vi "Trigger Ref DB (eFGV).vi"(7 "Action":T1, 8 "error in":errorcluster, 11 "Data In":bool) -> (0 "error out":errorcluster, 2 "ref":refnum<user-event>, 3 "Data out":bool)   [LabVIEW 2019]
uses:
  Controls/eFGV States.ctl
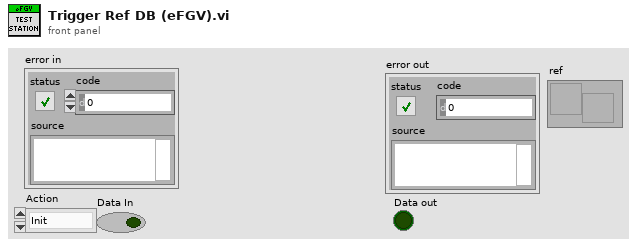
[diagram p1: front panel]
types:
  T1 = typedef "eFGV States.ctl" = enum16{"Init", "Read", "Write", "Exit"}
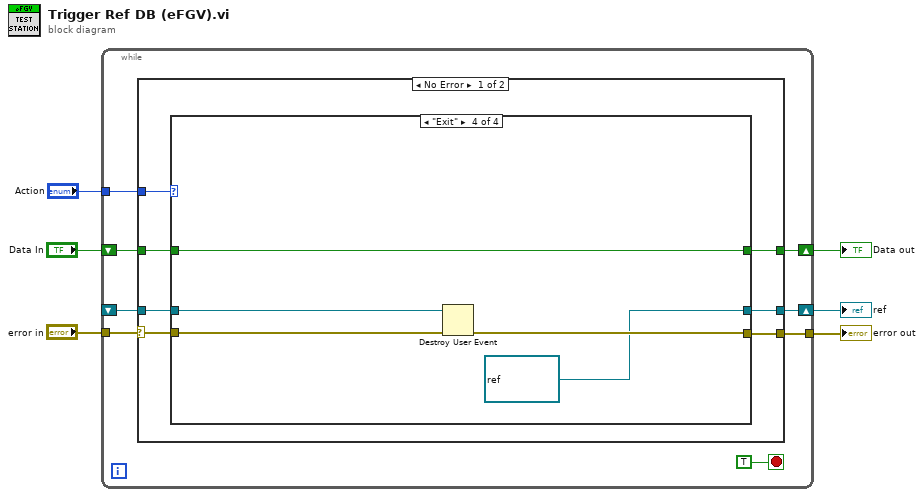
[diagram p0: block diagram]
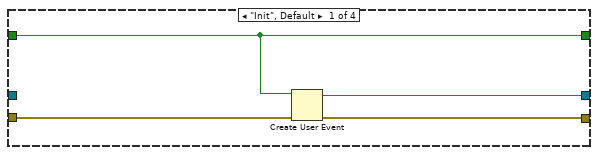
[diagram p2: hidden frame]
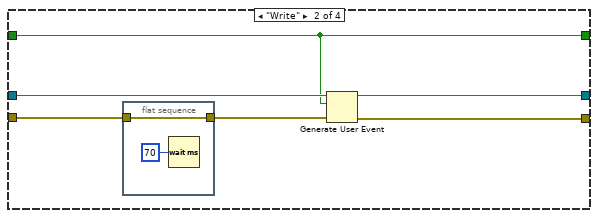
[diagram p3: hidden frame]
diagram:
  n1 = while {
    tunnel: "Action" -> [w11]
    tunnel: "error in" -> [w13]
    tunnel: [w12] -> w5
    shift-right: [w9] -> w2
    shift-left: "Data In" -> [w10]
    shift-right: [w8] -> w3
    shift-left: _ -> [w7]
    stop <- TRUE stop-if-true
    n2 = case shown="No Error" w13 {
      selector: w13 -> [w21 w42]
      tunnel: [w19 w42] -> w12
      tunnel: w11 -> [w20 _]
      tunnel: w10 -> [w18 w44]
      tunnel: [w17 w44] -> w9
      tunnel: [w16 w43] -> w8
      tunnel: w7 -> [w15 w43]
      frame No Error {
        n3 = case shown="\"Exit\"" w20 {
          tunnel: w21 -> [w25 w31 w35 w40]
          tunnel: [w24 w29 w35 w39] -> w19
          tunnel: w18 -> [w23 w26 w36 w41]
          tunnel: [w23 w26 w36 w41] -> w17
          tunnel: [w22 w27 w34 refnum<user-event> refnum ("Data In")] -> w16
          tunnel: w15 -> [_ w28 w34 w38]
          frame "Init", Default {
            n4 = Create User Event(user event datatype=w23, error in=w25) -> (user event=w22:refnum<user-event>, error out=w24:errorcluster)
          }
          frame "Write" {
            n5 = flat-sequence {
              tunnel: [w32] -> w30
              tunnel: w31 -> [w32]
              frame #0 {
                n6 = Wait (ms)(milliseconds to wait=u32 70) -> ()  [unwired: 1 out]
              }
            }
            n7 = Generate User Event(user event=w28, event data cluster=w26, error in=w30) -> (user event out=w27:refnum<user-event>, error out=w29:errorcluster)  [unwired: 1 in]
          }
          frame "Read" {
          }
          frame "Exit" {
            n8 = Destroy User Event(user event=w38, error in=w40) -> (error out=w39:errorcluster)
          }
        }
      }
      frame Error {
      }
    }
  }
  "error out" <- w5
  "ref" <- w3
  "Data out" <- w2
